vi "Parse New Activities.vi"(8 "error in (no error)":errorcluster, 10 "Club Activities JSON":string, 11 "Data Manager in":refnum<class "Data Manager.lvclass">) -> (0 "error out":errorcluster, 1 "History":T1={"Record Headers"=["Athlete", "Team", "Type", "Date", "Distance", "Moving Time", "Elapsed Time", "Total Elevation Gain"], "All Records"=[]}, 2 "Strava Club Activities":T2[](array[typedef]), 3 "Data Manager out":refnum<class "Data Manager.lvclass">)   [LabVIEW 2020, in "Data Manager.lvclass"]
uses:
  Data Manager.lvclass
  Strava JSON for Club Activities--cluster.ctl
  Data Manager.lvclass/Data Manager.ctl
  <vilib>/drjdpowell/SQLite Library/SQL Connection/Execute SQL (1D Integer results).vi
  <vilib>/drjdpowell/SQLite Library/SQLite.lvlib
  <vilib>/drjdpowell/SQLite Library/SQL Connection/Connection.lvclass
panel:
  out "index of element":i32
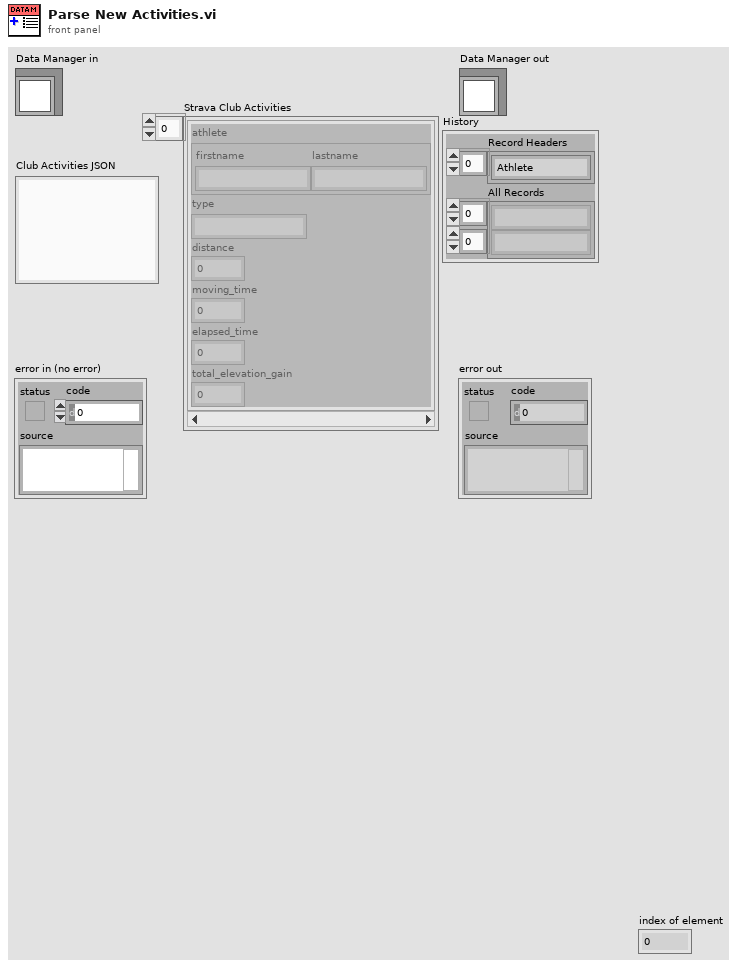
[diagram p1: front panel]
types:
  T1 = cluster{"Record Headers":string[], "All Records":string[][]}
  T2 = typedef "Data Manager.lvclass/Strava JSON for Club Activities--cluster.ctl" = cluster{"athlete":cluster{"firstname":string, "lastname":string}, "type":string, "distance":dbl, "moving_time":dbl, "elapsed_time":dbl, "total_elevation_gain":dbl}
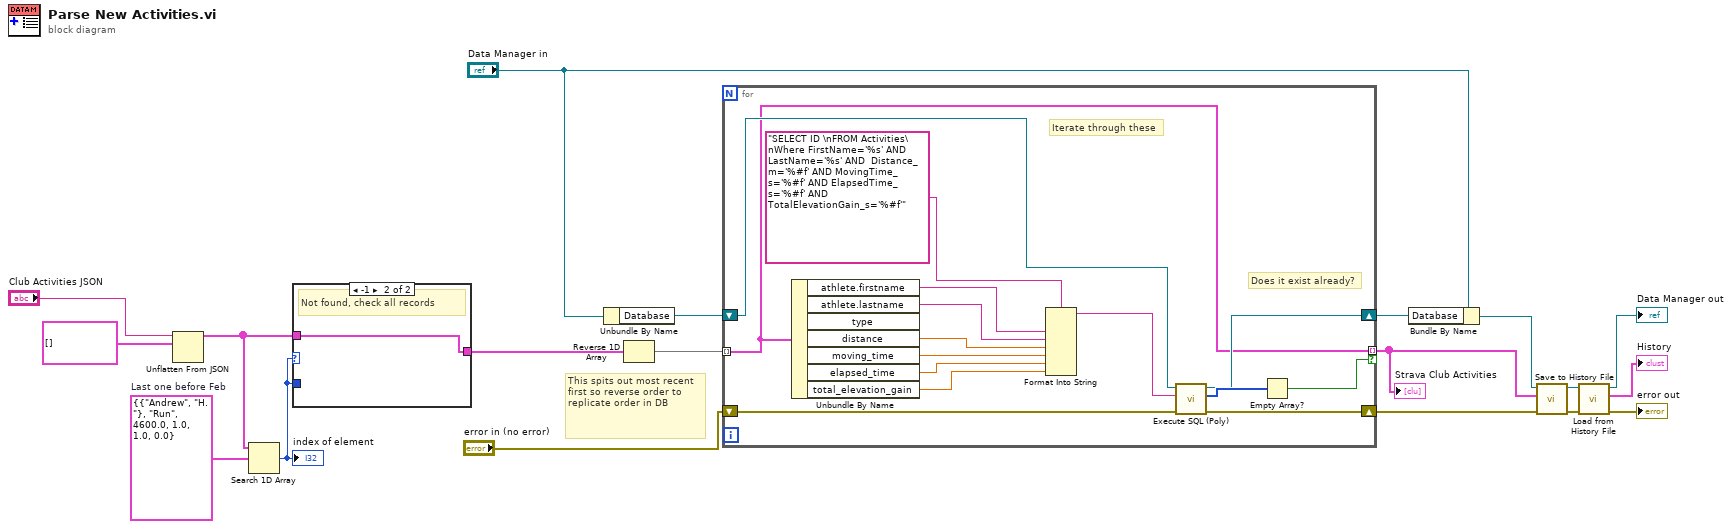
[diagram p0: block diagram]
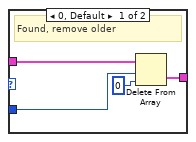
[diagram p2: hidden frame]
diagram:
  w19 = T2 {"athlete"={"firstname"="Andrew", "lastname"="H."}, "type"="Run", "distance"=4600.0, "moving_time"=1.0, "elapsed_time"=1.0, "total_elevation_gain"=0.0}  # Last one before Feb
  # "This spits out most recent first so reverse order to replicate order in DB"
  n1 = Unflatten From JSON(JSON string="Club Activities JSON", type and defaults=T2[] []) -> (value=w2:T2[])  [unwired: 5 in, 1 out]
  n2 = Search 1D Array(1D array=w2, element=w19) -> (index of element=w18:i32)  [unwired: 1 in]
  "index of element" <- w18
  n3 = case shown="-1" w18 {
    tunnel: w2 -> [w23 w24]
    tunnel: w18 -> [w22 _]
    tunnel: [w20 w24] -> w17
    frame 0, Default {
      # "Found, remove older"
      n4 = Delete From Array(array=w23, length=w22, index=0) -> (deleted portion=w20:T2[])  [unwired: 1 out]
    }
    frame -1 {
      # "Not found, check all records"
    }
  }
  n5 = Unbundle By Name("Data Manager in") -> ("Database"=w15:refnum<class "Connection.lvclass">)
  n6 = Reverse 1D Array(array=w17) -> (reversed array=w16:T2[])
  n7 = for {
    tunnel: w16 -> [w33] mode=indexing
    tunnel: [w33] -> w8 mode=indexing if=w38
    shift-right: [w36] -> w14
    shift-left: w15 -> [w37]
    shift-right: [w26] -> w5
    shift-left: "error in (no error)" -> [w25]
    # "Does it exist already?"
    # "Iterate through these"
    n8 = Unbundle By Name(w33) -> ("athlete.firstname"=w32:string, "athlete.lastname"=w31:string, "distance"=w30:dbl, "moving_time"=w29:dbl, "elapsed_time"=w28:dbl, "total_elevation_gain"=w27:dbl)  [unwired: 1 out]
    n9 = Format Into String(format string="SELECT ID \nFROM Activities\nWhere FirstName='%s' AND LastName='%s' AND  Distance_m='%#f' AND MovingTime_s='%#f' AND ElapsedTime_s='%#f' AND TotalElevationGain_s='%#f'" ("SQL"), w32, w31, w30, w29, w28, w27) -> (resulting string=w34:string)  [unwired: 2 in, 1 out]
    n10 = call-poly <vilib>:"Execute SQL (Poly).vi"("error in (no error)"=w25, "SQL"=w34, "SQLite Connection in"=w37) -> ("error out"=w26:errorcluster, "Result Set"=w39:i64[], "SQLite Connection"=w36:refnum<class "Connection.lvclass">)  [unwired: 5 in, 1 out]
    n11 = Empty Array?(array=w39) -> (empty?=w38:bool)
  }
  "Strava Club Activities" <- w8
  n12 = Bundle By Name(cluster="Data Manager in", "Database"=w14) -> (w12:refnum<class "Data Manager.lvclass">)
  n13 = call-dynamic "Save to History File.vi"("error in (no error)"=w5, "Records"=w8, "Data Manager in"=w12) -> ("error out"=w11:errorcluster, "Data Manager out"=w10:refnum<class "Data Manager.lvclass">)  [unwired: 7 in]
  n14 = call-dynamic "Load from History File.vi"("error in (no error)"=w11, "Data Manager in"=w10) -> ("error out"=→"error out":errorcluster, "History"=→"History":T1, "Data Manager out"=→"Data Manager out":refnum<class "Data Manager.lvclass">)  [unwired: 7 in]
